vi "Resistance Range.vi"(0 "VISA resource name":refnum<visa-resource-name>, 5 "Channel (1)":i32=1 min=1 max=16 step=1, 11 "error in (no error)":errorcluster) -> (3 "Autorange":bool, 4 "VISA resource name out":refnum<visa-resource-name>, 6 "Excitation Mode":u16(ring) items=["Voltage", "Current"], 8 "Excitation Range":u16(ring)=11 items=["2.00 uV / 1.00 pA", "6.32 uV / 3.16 pA", "20.0 uV / 10.0 pA", "63.2 uV / 31.6 pA", "200 uV / 100 pA", "632 uV / 316 pA", "2.00 mV / 1.00 nA", "6.32 mV / 3.16 nA", "20.0 mV / 10.0 nA", "63.2 mV / 31.6 nA", "200 mV / 100 nA", "632 mV / 316 nA", "1.00 uA", "3.16 uA", "10.0 uA", "31.6 uA", "100 uA", "316 uA", "1.00 mA", "3.16 mA", "10.0 mA", "31.6 mA"], 10 "Resistance Range":u16(ring)=21 items=["2.00 mOhm", "6.32 mOhm", "20.0 mOhm", "63.2 mOhm", "200 mOhm", "632 mOhm", "2.00 Ohm", "6.32 Ohm", "20.0 Ohm", "63.2 Ohm", "200 Ohm", "632 Ohm", "2.00 kOhm", "6.32 kOhm", "20.0 kOhm", "63.2 kOhm", "200 kOhm", "632 kOhm", "2.00 MOhm", "6.32 MOhm", "20.0 MOhm", "63.2 MOhm"], 14 "Excitation":bool=TRUE, 15 "error out":errorcluster)   [LabVIEW 2019, in "Lake Shore Cryotronics 370.lvlib"]
doc: "This VI queries the Excitation Modes, Resistance Range, and Autorange."
uses:
  Lake Shore Cryotronics 370.lvlib
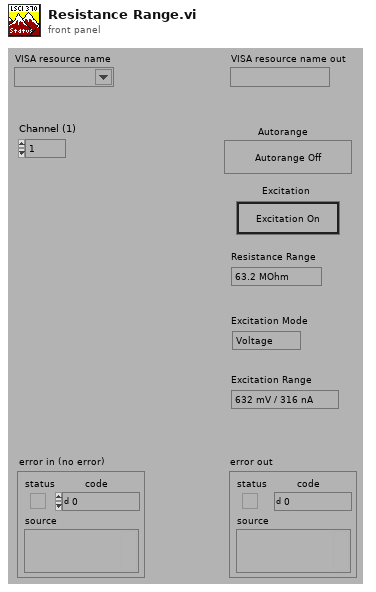
[diagram p1: front panel]
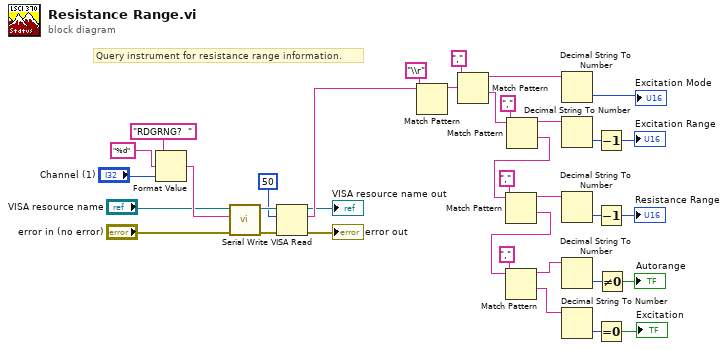
[diagram p0: block diagram]
diagram:
  # "Query instrument for resistance range information."
  n1 = Format Value(string ("")="RDGRNG?  ", format string="%d", value (0)="Channel (1)") -> (output string=w26:string)
  n2 = call "Serial Write.vi"("error in (no error)"="error in (no error)", "Write Buffer (\"\")"=w26, "VISA resource name"="VISA resource name") -> ("error out"=w34:errorcluster, "VISA resource name out"=w35:refnum<visa-resource-name>)  [unwired: 6 in, 1 out]
  n3 = VISA Read(VISA resource name=w35, byte count=50, error in (no error)=w34) -> (VISA resource name out=→"VISA resource name out":refnum<visa-resource-name>, read buffer=w32:string, error out=→"error out":errorcluster)  [unwired: 1 out]
  n4 = Match Pattern(string=w32, regular expression="\\r") -> (before substring=w29:string)  [unwired: 1 in, 3 out]
  n5 = Match Pattern(string=w29, regular expression=",") -> (before substring=w28:string, after substring=w18:string)  [unwired: 1 in, 2 out]
  n6 = Match Pattern(string=w18, regular expression=",") -> (before substring=w17:string, after substring=w14:string)  [unwired: 1 in, 2 out]
  n7 = Match Pattern(string=w14, regular expression=",") -> (before substring=w13:string, after substring=w10:string)  [unwired: 1 in, 2 out]
  n8 = Match Pattern(string=w10, regular expression=",") -> (before substring=w7:string, after substring=w6:string)  [unwired: 1 in, 2 out]
  n9 = Decimal String To Number(string=w28) -> (number=→"Excitation Mode":i32)  [unwired: 2 in, 1 out]
  n10 = Decimal String To Number(string=w17) -> (number=w16:i32)  [unwired: 2 in, 1 out]
  n11 = Decimal String To Number(string=w13) -> (number=w12:i32)  [unwired: 2 in, 1 out]
  n12 = Decimal String To Number(string=w7) -> (number=w9:i32)  [unwired: 2 in, 1 out]
  n13 = Decimal String To Number(string=w6) -> (number=w2:i32)  [unwired: 2 in, 1 out]
  n14 = Decrement(x=w16) -> (x-1=→"Excitation Range":i32)
  n15 = Decrement(x=w12) -> (x-1=→"Resistance Range":i32)
  n16 = Equal To 0?(x=w2) -> (x = 0?=→"Excitation":bool)
  n17 = Not Equal To 0?(x=w9) -> (x != 0?=→"Autorange":bool)
